vi "main(Test DQMH modules).bak.vi"() -> ()   [LabVIEW 2018, in "Application.lvlib"] (continued)
        n1621 = call "progress string(SubVI).vi"("String 3"=w3805, "String in"=w3806) -> ("String out"=w3807:string)  [unwired: 9 in]
        n1622 = call "FGV Driver Data.vi"("DUT index(1-60)"=w3804) -> ("DUT SC"=w3803:bool)  [unwired: 7 in, 3 out]
        n1623 = case shown="False" w3803 {
          tunnel: [w3832 _] -> w3812
          tunnel: w3809 -> [w3831 _]
          frame False {
            w3819 = T11 {"command"="", "command data"=variant} ("element")
            w3818 = "MEAS.mux6_1"
            n1624 = To Variant(anything=T4."mux6-1_channel0" ("mux6_1(3wires)_encode")) -> (Variant=w3817:variant)
            n1625 = To Variant(anything=T4."mux6_1_channel3_3" ("mux6_1(3wires)_encode")) -> (Variant=w3829:variant)
            n1626 = To Variant(anything=T4."mux6_1_channel3_2" ("mux6_1(3wires)_encode")) -> (Variant=w3827:variant)
            n1627 = Bundle By Name(cluster=w3819, "command"=w3818, "command data"=w3827) -> (w3826:T11)
            n1628 = Bundle By Name(cluster=w3819, "command"=w3818, "command data"=w3829) -> (w3825:T11)
            n1629 = Bundle By Name(cluster=w3819, "command"=w3818, "command data"=w3817) -> ()  [unwired: 1 out]
            n1630 = Bundle By Name(cluster=w3819, "command"="MEAS.DMM dual read") -> (w3823:T11)
            n1631 = Build Array(w3826, w3825, w3823) -> (w3821:T11[])
            n1632 = Reverse 1D Array(array=w3821) -> (reversed array=w3822:T11[])
            n1633 = for {
              tunnel: [w3838] -> w3832 mode=indexing
              tunnel: w3831 -> [w3837]
              tunnel: w3822 -> [w3836] mode=indexing
              n1634 = Unbundle By Name(w3836) -> ("command"=w3835:string, "command data"=w3834:variant)
              n1635 = call "App enquece.vi"("Priority Enquece"=TRUE, "command data"=w3834, "command"=w3835, "queue in"=w3837) -> ("error out"=w3838:errorcluster)  [unwired: 6 in, 1 out]
            }
          }
          frame True {
          }
        }
        n1636 = Merge Errors(w3810, w3812) -> (w3811:errorcluster)
      }
      frame "Test DRV 16" {
        w3845 = 16  # DUT index(0-59)
        n1637 = disable-structure shown="LOGGING==TRUE" {
          disable-tunnel: w3846 -> [w3881 _]
          frame condition #0 (active) {
            n1638 = Empty String/Path?(string/path=w3881) -> (empty?=w3884:bool)
            n1639 = Select(t="Quece timeout", s=w3884, f=w3881) -> (s? t:f=w3880:string)
            n1640 = call "string log (SubVI).vi"("Enum"=enum16{"Init", "Log", "Read"}."Log", "state Name"=w3880) -> ()  [unwired: 8 in, 2 out]
          }
          frame condition #1 {
          }
        }
        n1641 = call "progress string(SubVI).vi"("String 3"=w3846, "String in"=w3847) -> ("String out"=w3848:string)  [unwired: 9 in]
        n1642 = call "FGV Driver Data.vi"("DUT index(1-60)"=w3845) -> ("DUT SC"=w3844:bool)  [unwired: 7 in, 3 out]
        n1643 = case shown="False" w3844 {
          tunnel: [w3873 _] -> w3853
          tunnel: w3850 -> [w3872 _]
          frame False {
            w3860 = T11 {"command"="", "command data"=variant} ("element")
            w3859 = "MEAS.mux6_1"
            n1644 = To Variant(anything=T4."mux6-1_channel0" ("mux6_1(3wires)_encode")) -> (Variant=w3858:variant)
            n1645 = To Variant(anything=T4."mux6_1_channel4_3" ("mux6_1(3wires)_encode")) -> (Variant=w3870:variant)
            n1646 = To Variant(anything=T4."mux6_1_channel4_2" ("mux6_1(3wires)_encode")) -> (Variant=w3868:variant)
            n1647 = Bundle By Name(cluster=w3860, "command"=w3859, "command data"=w3868) -> (w3867:T11)
            n1648 = Bundle By Name(cluster=w3860, "command"=w3859, "command data"=w3870) -> (w3866:T11)
            n1649 = Bundle By Name(cluster=w3860, "command"=w3859, "command data"=w3858) -> ()  [unwired: 1 out]
            n1650 = Bundle By Name(cluster=w3860, "command"="MEAS.DMM dual read") -> (w3864:T11)
            n1651 = Build Array(w3867, w3866, w3864) -> (w3862:T11[])
            n1652 = Reverse 1D Array(array=w3862) -> (reversed array=w3863:T11[])
            n1653 = for {
              tunnel: [w3879] -> w3873 mode=indexing
              tunnel: w3872 -> [w3878]
              tunnel: w3863 -> [w3877] mode=indexing
              n1654 = Unbundle By Name(w3877) -> ("command"=w3876:string, "command data"=w3875:variant)
              n1655 = call "App enquece.vi"("Priority Enquece"=TRUE, "command data"=w3875, "command"=w3876, "queue in"=w3878) -> ("error out"=w3879:errorcluster)  [unwired: 6 in, 1 out]
            }
          }
          frame True {
          }
        }
        n1656 = Merge Errors(w3851, w3853) -> (w3852:errorcluster)
      }
      frame "Test DRV 17" {
        w3885 = 17  # DUT index(0-59)
        n1657 = disable-structure shown="LOGGING==TRUE" {
          disable-tunnel: w3887 -> [w3922 _]
          frame condition #0 (active) {
            n1658 = Empty String/Path?(string/path=w3922) -> (empty?=w3925:bool)
            n1659 = Select(t="Quece timeout", s=w3925, f=w3922) -> (s? t:f=w3921:string)
            n1660 = call "string log (SubVI).vi"("Enum"=enum16{"Init", "Log", "Read"}."Log", "state Name"=w3921) -> ()  [unwired: 8 in, 2 out]
          }
          frame condition #1 {
          }
        }
        n1661 = call "progress string(SubVI).vi"("String 3"=w3887, "String in"=w3888) -> ("String out"=w3889:string)  [unwired: 9 in]
        n1662 = call "FGV Driver Data.vi"("DUT index(1-60)"=w3885) -> ("DUT SC"=w3886:bool)  [unwired: 7 in, 3 out]
        n1663 = case shown="False" w3886 {
          tunnel: [w3914 _] -> w3894
          tunnel: w3891 -> [w3913 _]
          frame False {
            w3901 = T11 {"command"="", "command data"=variant} ("element")
            w3900 = "MEAS.mux6_1"
            n1664 = To Variant(anything=T4."mux6-1_channel0" ("mux6_1(3wires)_encode")) -> (Variant=w3899:variant)
            n1665 = To Variant(anything=T4."mux6_1_channel5_3" ("mux6_1(3wires)_encode")) -> (Variant=w3911:variant)
            n1666 = To Variant(anything=T4."mux6_1_channel5_2" ("mux6_1(3wires)_encode")) -> (Variant=w3909:variant)
            n1667 = Bundle By Name(cluster=w3901, "command"=w3900, "command data"=w3909) -> (w3908:T11)
            n1668 = Bundle By Name(cluster=w3901, "command"=w3900, "command data"=w3911) -> (w3907:T11)
            n1669 = Bundle By Name(cluster=w3901, "command"=w3900, "command data"=w3899) -> ()  [unwired: 1 out]
            n1670 = Bundle By Name(cluster=w3901, "command"="MEAS.DMM dual read") -> (w3905:T11)
            n1671 = Build Array(w3908, w3907, w3905) -> (w3903:T11[])
            n1672 = Reverse 1D Array(array=w3903) -> (reversed array=w3904:T11[])
            n1673 = for {
              tunnel: [w3920] -> w3914 mode=indexing
              tunnel: w3913 -> [w3919]
              tunnel: w3904 -> [w3918] mode=indexing
              n1674 = Unbundle By Name(w3918) -> ("command"=w3917:string, "command data"=w3916:variant)
              n1675 = call "App enquece.vi"("Priority Enquece"=TRUE, "command data"=w3916, "command"=w3917, "queue in"=w3919) -> ("error out"=w3920:errorcluster)  [unwired: 6 in, 1 out]
            }
          }
          frame True {
          }
        }
        n1676 = Merge Errors(w3892, w3894) -> (w3893:errorcluster)
      }
      frame "Test DRV 18" {
        w3929 = 18  # DUT index(0-59)
        n1677 = disable-structure shown="LOGGING==TRUE" {
          disable-tunnel: w3926 -> [w3963 _]
          frame condition #0 (active) {
            n1678 = Empty String/Path?(string/path=w3963) -> (empty?=w3966:bool)
            n1679 = Select(t="Quece timeout", s=w3966, f=w3963) -> (s? t:f=w3962:string)
            n1680 = call "string log (SubVI).vi"("Enum"=enum16{"Init", "Log", "Read"}."Log", "state Name"=w3962) -> ()  [unwired: 8 in, 2 out]
          }
          frame condition #1 {
          }
        }
        n1681 = call "progress string(SubVI).vi"("String 3"=w3926, "String in"=w3927) -> ("String out"=w3928:string)  [unwired: 9 in]
        n1682 = call "FGV Driver Data.vi"("DUT index(1-60)"=w3929) -> ("DUT SC"=w3930:bool)  [unwired: 7 in, 3 out]
        n1683 = case shown="False" w3930 {
          tunnel: [w3955 _] -> w3935
          tunnel: w3932 -> [w3954 _]
          frame False {
            w3942 = T11 {"command"="", "command data"=variant} ("element")
            w3941 = "MEAS.mux6_1"
            n1684 = To Variant(anything=T4."mux6-1_channel0" ("mux6_1(3wires)_encode")) -> (Variant=w3940:variant)
            n1685 = To Variant(anything=T4."mux6_1_channel6_3" ("mux6_1(3wires)_encode")) -> (Variant=w3952:variant)
            n1686 = To Variant(anything=T4."mux6_1_channel6_2" ("mux6_1(3wires)_encode")) -> (Variant=w3950:variant)
            n1687 = Bundle By Name(cluster=w3942, "command"=w3941, "command data"=w3950) -> (w3949:T11)
            n1688 = Bundle By Name(cluster=w3942, "command"=w3941, "command data"=w3952) -> (w3948:T11)
            n1689 = Bundle By Name(cluster=w3942, "command"=w3941, "command data"=w3940) -> ()  [unwired: 1 out]
            n1690 = Bundle By Name(cluster=w3942, "command"="MEAS.DMM dual read") -> (w3946:T11)
            n1691 = Build Array(w3949, w3948, w3946) -> (w3944:T11[])
            n1692 = Reverse 1D Array(array=w3944) -> (reversed array=w3945:T11[])
            n1693 = for {
              tunnel: [w3961] -> w3955 mode=indexing
              tunnel: w3954 -> [w3960]
              tunnel: w3945 -> [w3959] mode=indexing
              n1694 = Unbundle By Name(w3959) -> ("command"=w3958:string, "command data"=w3957:variant)
              n1695 = call "App enquece.vi"("Priority Enquece"=TRUE, "command data"=w3957, "command"=w3958, "queue in"=w3960) -> ("error out"=w3961:errorcluster)  [unwired: 6 in, 1 out]
            }
          }
          frame True {
          }
        }
        n1696 = Merge Errors(w3933, w3935) -> (w3934:errorcluster)
      }
      frame "Test DRV 19" {
        w3968 = 19  # DUT index(0-59)
        n1697 = disable-structure shown="LOGGING==TRUE" {
          disable-tunnel: w3969 -> [w4004 _]
          frame condition #0 (active) {
            n1698 = Empty String/Path?(string/path=w4004) -> (empty?=w4007:bool)
            n1699 = Select(t="Quece timeout", s=w4007, f=w4004) -> (s? t:f=w4003:string)
            n1700 = call "string log (SubVI).vi"("Enum"=enum16{"Init", "Log", "Read"}."Log", "state Name"=w4003) -> ()  [unwired: 8 in, 2 out]
          }
          frame condition #1 {
          }
        }
        n1701 = call "progress string(SubVI).vi"("String 3"=w3969, "String in"=w3970) -> ("String out"=w3971:string)  [unwired: 9 in]
        n1702 = call "FGV Driver Data.vi"("DUT index(1-60)"=w3968) -> ("DUT SC"=w3967:bool)  [unwired: 7 in, 3 out]
        n1703 = case shown="False" w3967 {
          tunnel: [w3996 _] -> w3976
          tunnel: w3973 -> [w3995 _]
          frame False {
            w3983 = T11 {"command"="", "command data"=variant} ("element")
            w3982 = "MEAS.mux6_1"
            n1704 = To Variant(anything=T4."mux6-1_channel0" ("mux6_1(3wires)_encode")) -> (Variant=w3981:variant)
            n1705 = To Variant(anything=T4."mux6_1_channel1_3" ("mux6_1(3wires)_encode")) -> (Variant=w3993:variant)
            n1706 = To Variant(anything=T4."mux6-1_channel1_2" ("mux6_1(3wires)_encode")) -> (Variant=w3991:variant)
            n1707 = Bundle By Name(cluster=w3983, "command"=w3982, "command data"=w3991) -> (w3990:T11)
            n1708 = Bundle By Name(cluster=w3983, "command"=w3982, "command data"=w3993) -> (w3989:T11)
            n1709 = Bundle By Name(cluster=w3983, "command"=w3982, "command data"=w3981) -> ()  [unwired: 1 out]
            n1710 = Bundle By Name(cluster=w3983, "command"="MEAS.DMM dual read") -> (w3987:T11)
            n1711 = Build Array(w3990, w3989, w3987) -> (w3985:T11[])
            n1712 = Reverse 1D Array(array=w3985) -> (reversed array=w3986:T11[])
            n1713 = for {
              tunnel: [w4002] -> w3996 mode=indexing
              tunnel: w3995 -> [w4001]
              tunnel: w3986 -> [w4000] mode=indexing
              n1714 = Unbundle By Name(w4000) -> ("command"=w3999:string, "command data"=w3998:variant)
              n1715 = call "App enquece.vi"("Priority Enquece"=TRUE, "command data"=w3998, "command"=w3999, "queue in"=w4001) -> ("error out"=w4002:errorcluster)  [unwired: 6 in, 1 out]
            }
          }
          frame True {
          }
        }
        n1716 = Merge Errors(w3974, w3976) -> (w3975:errorcluster)
      }
      frame "Test DRV 20" {
        w4009 = 20  # DUT index(0-59)
        n1717 = disable-structure shown="LOGGING==TRUE" {
          disable-tunnel: w4010 -> [w4045 _]
          frame condition #0 (active) {
            n1718 = Empty String/Path?(string/path=w4045) -> (empty?=w4048:bool)
            n1719 = Select(t="Quece timeout", s=w4048, f=w4045) -> (s? t:f=w4044:string)
            n1720 = call "string log (SubVI).vi"("Enum"=enum16{"Init", "Log", "Read"}."Log", "state Name"=w4044) -> ()  [unwired: 8 in, 2 out]
          }
          frame condition #1 {
          }
        }
        n1721 = call "progress string(SubVI).vi"("String 3"=w4010, "String in"=w4011) -> ("String out"=w4012:string)  [unwired: 9 in]
        n1722 = call "FGV Driver Data.vi"("DUT index(1-60)"=w4009) -> ("DUT SC"=w4008:bool)  [unwired: 7 in, 3 out]
        n1723 = case shown="False" w4008 {
          tunnel: [w4037 _] -> w4017
          tunnel: w4014 -> [w4036 _]
          frame False {
            w4024 = T11 {"command"="", "command data"=variant} ("element")
            w4023 = "MEAS.mux6_1"
            n1724 = To Variant(anything=T4."mux6-1_channel0" ("mux6_1(3wires)_encode")) -> (Variant=w4022:variant)
            n1725 = To Variant(anything=T4."mux6_1_channel2_3" ("mux6_1(3wires)_encode")) -> (Variant=w4034:variant)
            n1726 = To Variant(anything=T4."mux6_1_channel2_2" ("mux6_1(3wires)_encode")) -> (Variant=w4032:variant)
            n1727 = Bundle By Name(cluster=w4024, "command"=w4023, "command data"=w4032) -> (w4031:T11)
            n1728 = Bundle By Name(cluster=w4024, "command"=w4023, "command data"=w4034) -> (w4030:T11)
            n1729 = Bundle By Name(cluster=w4024, "command"=w4023, "command data"=w4022) -> ()  [unwired: 1 out]
            n1730 = Bundle By Name(cluster=w4024, "command"="MEAS.DMM dual read") -> (w4028:T11)
            n1731 = Build Array(w4031, w4030, w4028) -> (w4026:T11[])
            n1732 = Reverse 1D Array(array=w4026) -> (reversed array=w4027:T11[])
            n1733 = for {
              tunnel: [w4043] -> w4037 mode=indexing
              tunnel: w4036 -> [w4042]
              tunnel: w4027 -> [w4041] mode=indexing
              n1734 = Unbundle By Name(w4041) -> ("command"=w4040:string, "command data"=w4039:variant)
              n1735 = call "App enquece.vi"("Priority Enquece"=TRUE, "command data"=w4039, "command"=w4040, "queue in"=w4042) -> ("error out"=w4043:errorcluster)  [unwired: 6 in, 1 out]
            }
          }
          frame True {
          }
        }
        n1736 = Merge Errors(w4015, w4017) -> (w4016:errorcluster)
      }
      frame "Test DRV 21" {
        w4050 = 21  # DUT index(0-59)
        n1737 = disable-structure shown="LOGGING==TRUE" {
          disable-tunnel: w4051 -> [w4086 _]
          frame condition #0 (active) {
            n1738 = Empty String/Path?(string/path=w4086) -> (empty?=w4089:bool)
            n1739 = Select(t="Quece timeout", s=w4089, f=w4086) -> (s? t:f=w4085:string)
            n1740 = call "string log (SubVI).vi"("Enum"=enum16{"Init", "Log", "Read"}."Log", "state Name"=w4085) -> ()  [unwired: 8 in, 2 out]
          }
          frame condition #1 {
          }
        }
        n1741 = call "progress string(SubVI).vi"("String 3"=w4051, "String in"=w4052) -> ("String out"=w4053:string)  [unwired: 9 in]
        n1742 = call "FGV Driver Data.vi"("DUT index(1-60)"=w4050) -> ("DUT SC"=w4049:bool)  [unwired: 7 in, 3 out]
        n1743 = case shown="False" w4049 {
          tunnel: [w4078 _] -> w4058
          tunnel: w4055 -> [w4077 _]
          frame False {
            w4065 = T11 {"command"="", "command data"=variant} ("element")
            w4064 = "MEAS.mux6_1"
            n1744 = To Variant(anything=T4."mux6-1_channel0" ("mux6_1(3wires)_encode")) -> (Variant=w4063:variant)
            n1745 = To Variant(anything=T4."mux6_1_channel3_3" ("mux6_1(3wires)_encode")) -> (Variant=w4075:variant)
            n1746 = To Variant(anything=T4."mux6_1_channel3_2" ("mux6_1(3wires)_encode")) -> (Variant=w4073:variant)
            n1747 = Bundle By Name(cluster=w4065, "command"=w4064, "command data"=w4073) -> (w4072:T11)
            n1748 = Bundle By Name(cluster=w4065, "command"=w4064, "command data"=w4075) -> (w4071:T11)
            n1749 = Bundle By Name(cluster=w4065, "command"=w4064, "command data"=w4063) -> ()  [unwired: 1 out]
            n1750 = Bundle By Name(cluster=w4065, "command"="MEAS.DMM dual read") -> (w4069:T11)
            n1751 = Build Array(w4072, w4071, w4069) -> (w4067:T11[])
            n1752 = Reverse 1D Array(array=w4067) -> (reversed array=w4068:T11[])
            n1753 = for {
              tunnel: [w4084] -> w4078 mode=indexing
              tunnel: w4077 -> [w4083]
              tunnel: w4068 -> [w4082] mode=indexing
              n1754 = Unbundle By Name(w4082) -> ("command"=w4081:string, "command data"=w4080:variant)
              n1755 = call "App enquece.vi"("Priority Enquece"=TRUE, "command data"=w4080, "command"=w4081, "queue in"=w4083) -> ("error out"=w4084:errorcluster)  [unwired: 6 in, 1 out]
            }
          }
          frame True {
          }
        }
        n1756 = Merge Errors(w4056, w4058) -> (w4057:errorcluster)
      }
      frame "Test DRV 22" {
        w4091 = 22  # DUT index(0-59)
        n1757 = disable-structure shown="LOGGING==TRUE" {
          disable-tunnel: w4092 -> [w4127 _]
          frame condition #0 (active) {
            n1758 = Empty String/Path?(string/path=w4127) -> (empty?=w4130:bool)
            n1759 = Select(t="Quece timeout", s=w4130, f=w4127) -> (s? t:f=w4126:string)
            n1760 = call "string log (SubVI).vi"("Enum"=enum16{"Init", "Log", "Read"}."Log", "state Name"=w4126) -> ()  [unwired: 8 in, 2 out]
          }
          frame condition #1 {
          }
        }
        n1761 = call "progress string(SubVI).vi"("String 3"=w4092, "String in"=w4093) -> ("String out"=w4094:string)  [unwired: 9 in]
        n1762 = call "FGV Driver Data.vi"("DUT index(1-60)"=w4091) -> ("DUT SC"=w4090:bool)  [unwired: 7 in, 3 out]
        n1763 = case shown="False" w4090 {
          tunnel: [w4119 _] -> w4099
          tunnel: w4096 -> [w4118 _]
          frame False {
            w4106 = T11 {"command"="", "command data"=variant} ("element")
            w4105 = "MEAS.mux6_1"
            n1764 = To Variant(anything=T4."mux6-1_channel0" ("mux6_1(3wires)_encode")) -> (Variant=w4104:variant)
            n1765 = To Variant(anything=T4."mux6_1_channel4_3" ("mux6_1(3wires)_encode")) -> (Variant=w4116:variant)
            n1766 = To Variant(anything=T4."mux6_1_channel4_2" ("mux6_1(3wires)_encode")) -> (Variant=w4114:variant)
            n1767 = Bundle By Name(cluster=w4106, "command"=w4105, "command data"=w4114) -> (w4113:T11)
            n1768 = Bundle By Name(cluster=w4106, "command"=w4105, "command data"=w4116) -> (w4112:T11)
            n1769 = Bundle By Name(cluster=w4106, "command"=w4105, "command data"=w4104) -> ()  [unwired: 1 out]
            n1770 = Bundle By Name(cluster=w4106, "command"="MEAS.DMM dual read") -> (w4110:T11)
            n1771 = Build Array(w4113, w4112, w4110) -> (w4108:T11[])
            n1772 = Reverse 1D Array(array=w4108) -> (reversed array=w4109:T11[])
            n1773 = for {
              tunnel: [w4125] -> w4119 mode=indexing
              tunnel: w4118 -> [w4124]
              tunnel: w4109 -> [w4123] mode=indexing
              n1774 = Unbundle By Name(w4123) -> ("command"=w4122:string, "command data"=w4121:variant)
              n1775 = call "App enquece.vi"("Priority Enquece"=TRUE, "command data"=w4121, "command"=w4122, "queue in"=w4124) -> ("error out"=w4125:errorcluster)  [unwired: 6 in, 1 out]
            }
          }
          frame True {
          }
        }
        n1776 = Merge Errors(w4097, w4099) -> (w4098:errorcluster)
      }
      frame "Test DRV 23" {
        w4132 = 23  # DUT index(0-59)
        n1777 = disable-structure shown="LOGGING==TRUE" {
          disable-tunnel: w4133 -> [w4168 _]
          frame condition #0 (active) {
            n1778 = Empty String/Path?(string/path=w4168) -> (empty?=w4171:bool)
            n1779 = Select(t="Quece timeout", s=w4171, f=w4168) -> (s? t:f=w4167:string)
            n1780 = call "string log (SubVI).vi"("Enum"=enum16{"Init", "Log", "Read"}."Log", "state Name"=w4167) -> ()  [unwired: 8 in, 2 out]
          }
          frame condition #1 {
          }
        }
        n1781 = call "progress string(SubVI).vi"("String 3"=w4133, "String in"=w4134) -> ("String out"=w4135:string)  [unwired: 9 in]
        n1782 = call "FGV Driver Data.vi"("DUT index(1-60)"=w4132) -> ("DUT SC"=w4131:bool)  [unwired: 7 in, 3 out]
        n1783 = case shown="False" w4131 {
          tunnel: [w4160 _] -> w4140
          tunnel: w4137 -> [w4159 _]
          frame False {
            w4147 = T11 {"command"="", "command data"=variant} ("element")
            w4146 = "MEAS.mux6_1"
            n1784 = To Variant(anything=T4."mux6-1_channel0" ("mux6_1(3wires)_encode")) -> (Variant=w4145:variant)
            n1785 = To Variant(anything=T4."mux6_1_channel5_3" ("mux6_1(3wires)_encode")) -> (Variant=w4157:variant)
            n1786 = To Variant(anything=T4."mux6_1_channel5_2" ("mux6_1(3wires)_encode")) -> (Variant=w4155:variant)
            n1787 = Bundle By Name(cluster=w4147, "command"=w4146, "command data"=w4155) -> (w4154:T11)
            n1788 = Bundle By Name(cluster=w4147, "command"=w4146, "command data"=w4157) -> (w4153:T11)
            n1789 = Bundle By Name(cluster=w4147, "command"=w4146, "command data"=w4145) -> ()  [unwired: 1 out]
            n1790 = Bundle By Name(cluster=w4147, "command"="MEAS.DMM dual read") -> (w4151:T11)
            n1791 = Build Array(w4154, w4153, w4151) -> (w4149:T11[])
            n1792 = Reverse 1D Array(array=w4149) -> (reversed array=w4150:T11[])
            n1793 = for {
              tunnel: [w4166] -> w4160 mode=indexing
              tunnel: w4159 -> [w4165]
              tunnel: w4150 -> [w4164] mode=indexing
              n1794 = Unbundle By Name(w4164) -> ("command"=w4163:string, "command data"=w4162:variant)
              n1795 = call "App enquece.vi"("Priority Enquece"=TRUE, "command data"=w4162, "command"=w4163, "queue in"=w4165) -> ("error out"=w4166:errorcluster)  [unwired: 6 in, 1 out]
            }
          }
          frame True {
          }
        }
        n1796 = Merge Errors(w4138, w4140) -> (w4139:errorcluster)
      }
      frame "Test DRV 24" {
        w4173 = 24  # DUT index(0-59)
        n1797 = disable-structure shown="LOGGING==TRUE" {
          disable-tunnel: w4174 -> [w4209 _]
          frame condition #0 (active) {
            n1798 = Empty String/Path?(string/path=w4209) -> (empty?=w4212:bool)
            n1799 = Select(t="Quece timeout", s=w4212, f=w4209) -> (s? t:f=w4208:string)
            n1800 = call "string log (SubVI).vi"("Enum"=enum16{"Init", "Log", "Read"}."Log", "state Name"=w4208) -> ()  [unwired: 8 in, 2 out]
          }
          frame condition #1 {
          }
        }
        n1801 = call "progress string(SubVI).vi"("String 3"=w4174, "String in"=w4175) -> ("String out"=w4176:string)  [unwired: 9 in]
        n1802 = call "FGV Driver Data.vi"("DUT index(1-60)"=w4173) -> ("DUT SC"=w4172:bool)  [unwired: 7 in, 3 out]
        n1803 = case shown="False" w4172 {
          tunnel: [w4201 _] -> w4181
          tunnel: w4178 -> [w4200 _]
          frame False {
            w4188 = T11 {"command"="", "command data"=variant} ("element")
            w4187 = "MEAS.mux6_1"
            n1804 = To Variant(anything=T4."mux6-1_channel0" ("mux6_1(3wires)_encode")) -> (Variant=w4186:variant)
            n1805 = To Variant(anything=T4."mux6_1_channel6_3" ("mux6_1(3wires)_encode")) -> (Variant=w4198:variant)
            n1806 = To Variant(anything=T4."mux6_1_channel6_2" ("mux6_1(3wires)_encode")) -> (Variant=w4196:variant)
            n1807 = Bundle By Name(cluster=w4188, "command"=w4187, "command data"=w4196) -> (w4195:T11)
            n1808 = Bundle By Name(cluster=w4188, "command"=w4187, "command data"=w4198) -> (w4194:T11)
            n1809 = Bundle By Name(cluster=w4188, "command"=w4187, "command data"=w4186) -> ()  [unwired: 1 out]
            n1810 = Bundle By Name(cluster=w4188, "command"="MEAS.DMM dual read") -> (w4192:T11)
            n1811 = Build Array(w4195, w4194, w4192) -> (w4190:T11[])
            n1812 = Reverse 1D Array(array=w4190) -> (reversed array=w4191:T11[])
            n1813 = for {
              tunnel: [w4207] -> w4201 mode=indexing
              tunnel: w4200 -> [w4206]
              tunnel: w4191 -> [w4205] mode=indexing
              n1814 = Unbundle By Name(w4205) -> ("command"=w4204:string, "command data"=w4203:variant)
              n1815 = call "App enquece.vi"("Priority Enquece"=TRUE, "command data"=w4203, "command"=w4204, "queue in"=w4206) -> ("error out"=w4207:errorcluster)  [unwired: 6 in, 1 out]
            }
          }
          frame True {
          }
        }
        n1816 = Merge Errors(w4179, w4181) -> (w4180:errorcluster)
      }
      frame "Test DRV 25" {
        w4214 = 25  # DUT index(0-59)
        n1817 = disable-structure shown="LOGGING==TRUE" {
          disable-tunnel: w4215 -> [w4250 _]
          frame condition #0 (active) {
            n1818 = Empty String/Path?(string/path=w4250) -> (empty?=w4253:bool)
            n1819 = Select(t="Quece timeout", s=w4253, f=w4250) -> (s? t:f=w4249:string)
            n1820 = call "string log (SubVI).vi"("Enum"=enum16{"Init", "Log", "Read"}."Log", "state Name"=w4249) -> ()  [unwired: 8 in, 2 out]
          }
          frame condition #1 {
          }
        }
        n1821 = call "progress string(SubVI).vi"("String 3"=w4215, "String in"=w4216) -> ("String out"=w4217:string)  [unwired: 9 in]
        n1822 = call "FGV Driver Data.vi"("DUT index(1-60)"=w4214) -> ("DUT SC"=w4213:bool)  [unwired: 7 in, 3 out]
        n1823 = case shown="False" w4213 {
          tunnel: [w4242 _] -> w4222
          tunnel: w4219 -> [w4241 _]
          frame False {
            w4229 = T11 {"command"="", "command data"=variant} ("element")
            w4228 = "MEAS.mux6_1"
            n1824 = To Variant(anything=T4."mux6-1_channel0" ("mux6_1(3wires)_encode")) -> (Variant=w4227:variant)
            n1825 = To Variant(anything=T4."mux6_1_channel1_3" ("mux6_1(3wires)_encode")) -> (Variant=w4239:variant)
            n1826 = To Variant(anything=T4."mux6-1_channel1_2" ("mux6_1(3wires)_encode")) -> (Variant=w4237:variant)
            n1827 = Bundle By Name(cluster=w4229, "command"=w4228, "command data"=w4237) -> (w4236:T11)
            n1828 = Bundle By Name(cluster=w4229, "command"=w4228, "command data"=w4239) -> (w4235:T11)
            n1829 = Bundle By Name(cluster=w4229, "command"=w4228, "command data"=w4227) -> ()  [unwired: 1 out]
            n1830 = Bundle By Name(cluster=w4229, "command"="MEAS.DMM dual read") -> (w4233:T11)
            n1831 = Build Array(w4236, w4235, w4233) -> (w4231:T11[])
            n1832 = Reverse 1D Array(array=w4231) -> (reversed array=w4232:T11[])
            n1833 = for {
              tunnel: [w4248] -> w4242 mode=indexing
              tunnel: w4241 -> [w4247]
              tunnel: w4232 -> [w4246] mode=indexing
              n1834 = Unbundle By Name(w4246) -> ("command"=w4245:string, "command data"=w4244:variant)
              n1835 = call "App enquece.vi"("Priority Enquece"=TRUE, "command data"=w4244, "command"=w4245, "queue in"=w4247) -> ("error out"=w4248:errorcluster)  [unwired: 6 in, 1 out]
            }
          }
          frame True {
          }
        }
        n1836 = Merge Errors(w4220, w4222) -> (w4221:errorcluster)
      }
      frame "Test DRV 26" {
        w4255 = 26  # DUT index(0-59)
        n1837 = disable-structure shown="LOGGING==TRUE" {
          disable-tunnel: w4256 -> [w4291 _]
          frame condition #0 (active) {
            n1838 = Empty String/Path?(string/path=w4291) -> (empty?=w4294:bool)
            n1839 = Select(t="Quece timeout", s=w4294, f=w4291) -> (s? t:f=w4290:string)
            n1840 = call "string log (SubVI).vi"("Enum"=enum16{"Init", "Log", "Read"}."Log", "state Name"=w4290) -> ()  [unwired: 8 in, 2 out]
          }
          frame condition #1 {
          }
        }
        n1841 = call "progress string(SubVI).vi"("String 3"=w4256, "String in"=w4257) -> ("String out"=w4258:string)  [unwired: 9 in]
        n1842 = call "FGV Driver Data.vi"("DUT index(1-60)"=w4255) -> ("DUT SC"=w4254:bool)  [unwired: 7 in, 3 out]
        n1843 = case shown="False" w4254 {
          tunnel: [w4283 _] -> w4263
          tunnel: w4260 -> [w4282 _]
          frame False {
            w4270 = T11 {"command"="", "command data"=variant} ("element")
            w4269 = "MEAS.mux6_1"
            n1844 = To Variant(anything=T4."mux6-1_channel0" ("mux6_1(3wires)_encode")) -> (Variant=w4268:variant)
            n1845 = To Variant(anything=T4."mux6_1_channel2_3" ("mux6_1(3wires)_encode")) -> (Variant=w4280:variant)
            n1846 = To Variant(anything=T4."mux6_1_channel2_2" ("mux6_1(3wires)_encode")) -> (Variant=w4278:variant)
            n1847 = Bundle By Name(cluster=w4270, "command"=w4269, "command data"=w4278) -> (w4277:T11)
            n1848 = Bundle By Name(cluster=w4270, "command"=w4269, "command data"=w4280) -> (w4276:T11)
            n1849 = Bundle By Name(cluster=w4270, "command"=w4269, "command data"=w4268) -> ()  [unwired: 1 out]
            n1850 = Bundle By Name(cluster=w4270, "command"="MEAS.DMM dual read") -> (w4274:T11)
            n1851 = Build Array(w4277, w4276, w4274) -> (w4272:T11[])
            n1852 = Reverse 1D Array(array=w4272) -> (reversed array=w4273:T11[])
            n1853 = for {
              tunnel: [w4289] -> w4283 mode=indexing
              tunnel: w4282 -> [w4288]
              tunnel: w4273 -> [w4287] mode=indexing
              n1854 = Unbundle By Name(w4287) -> ("command"=w4286:string, "command data"=w4285:variant)
              n1855 = call "App enquece.vi"("Priority Enquece"=TRUE, "command data"=w4285, "command"=w4286, "queue in"=w4288) -> ("error out"=w4289:errorcluster)  [unwired: 6 in, 1 out]
            }
          }
          frame True {
          }
        }
        n1856 = Merge Errors(w4261, w4263) -> (w4262:errorcluster)
      }
      frame "Test DRV 27" {
        w4296 = 27  # DUT index(0-59)
        n1857 = disable-structure shown="LOGGING==TRUE" {
          disable-tunnel: w4297 -> [w4332 _]
          frame condition #0 (active) {
            n1858 = Empty String/Path?(string/path=w4332) -> (empty?=w4335:bool)
            n1859 = Select(t="Quece timeout", s=w4335, f=w4332) -> (s? t:f=w4331:string)
            n1860 = call "string log (SubVI).vi"("Enum"=enum16{"Init", "Log", "Read"}."Log", "state Name"=w4331) -> ()  [unwired: 8 in, 2 out]
          }
          frame condition #1 {
          }
        }
        n1861 = call "progress string(SubVI).vi"("String 3"=w4297, "String in"=w4298) -> ("String out"=w4299:string)  [unwired: 9 in]
        n1862 = call "FGV Driver Data.vi"("DUT index(1-60)"=w4296) -> ("DUT SC"=w4295:bool)  [unwired: 7 in, 3 out]
        n1863 = case shown="False" w4295 {
          tunnel: [w4324 _] -> w4304
          tunnel: w4301 -> [w4323 _]
          frame False {
            w4311 = T11 {"command"="", "command data"=variant} ("element")
            w4310 = "MEAS.mux6_1"
            n1864 = To Variant(anything=T4."mux6-1_channel0" ("mux6_1(3wires)_encode")) -> (Variant=w4309:variant)
            n1865 = To Variant(anything=T4."mux6_1_channel3_3" ("mux6_1(3wires)_encode")) -> (Variant=w4321:variant)
            n1866 = To Variant(anything=T4."mux6_1_channel3_2" ("mux6_1(3wires)_encode")) -> (Variant=w4319:variant)
            n1867 = Bundle By Name(cluster=w4311, "command"=w4310, "command data"=w4319) -> (w4318:T11)
            n1868 = Bundle By Name(cluster=w4311, "command"=w4310, "command data"=w4321) -> (w4317:T11)
            n1869 = Bundle By Name(cluster=w4311, "command"=w4310, "command data"=w4309) -> ()  [unwired: 1 out]
            n1870 = Bundle By Name(cluster=w4311, "command"="MEAS.DMM dual read") -> (w4315:T11)
            n1871 = Build Array(w4318, w4317, w4315) -> (w4313:T11[])
            n1872 = Reverse 1D Array(array=w4313) -> (reversed array=w4314:T11[])
            n1873 = for {
              tunnel: [w4330] -> w4324 mode=indexing
              tunnel: w4323 -> [w4329]
              tunnel: w4314 -> [w4328] mode=indexing
              n1874 = Unbundle By Name(w4328) -> ("command"=w4327:string, "command data"=w4326:variant)
              n1875 = call "App enquece.vi"("Priority Enquece"=TRUE, "command data"=w4326, "command"=w4327, "queue in"=w4329) -> ("error out"=w4330:errorcluster)  [unwired: 6 in, 1 out]
            }
          }
          frame True {
          }
        }
        n1876 = Merge Errors(w4302, w4304) -> (w4303:errorcluster)
      }
      frame "Test DRV 28" {
        w4337 = 28  # DUT index(0-59)
        n1877 = disable-structure shown="LOGGING==TRUE" {
          disable-tunnel: w4338 -> [w4373 _]
          frame condition #0 (active) {
            n1878 = Empty String/Path?(string/path=w4373) -> (empty?=w4376:bool)
            n1879 = Select(t="Quece timeout", s=w4376, f=w4373) -> (s? t:f=w4372:string)
            n1880 = call "string log (SubVI).vi"("Enum"=enum16{"Init", "Log", "Read"}."Log", "state Name"=w4372) -> ()  [unwired: 8 in, 2 out]
          }
          frame condition #1 {
          }
        }
        n1881 = call "progress string(SubVI).vi"("String 3"=w4338, "String in"=w4339) -> ("String out"=w4340:string)  [unwired: 9 in]
        n1882 = call "FGV Driver Data.vi"("DUT index(1-60)"=w4337) -> ("DUT SC"=w4336:bool)  [unwired: 7 in, 3 out]
        n1883 = case shown="False" w4336 {
          tunnel: [w4365 _] -> w4345
          tunnel: w4342 -> [w4364 _]
          frame False {
            w4350 = T11 {"command"="", "command data"=variant} ("element")
            w4352 = "MEAS.mux6_1"
            n1884 = To Variant(anything=T4."mux6-1_channel0" ("mux6_1(3wires)_encode")) -> (Variant=w4351:variant)
            n1885 = To Variant(anything=T4."mux6_1_channel4_3" ("mux6_1(3wires)_encode")) -> (Variant=w4362:variant)
            n1886 = To Variant(anything=T4."mux6_1_channel4_2" ("mux6_1(3wires)_encode")) -> (Variant=w4360:variant)
            n1887 = Bundle By Name(cluster=w4350, "command"=w4352, "command data"=w4360) -> (w4359:T11)
            n1888 = Bundle By Name(cluster=w4350, "command"=w4352, "command data"=w4362) -> (w4358:T11)
            n1889 = Bundle By Name(cluster=w4350, "command"=w4352, "command data"=w4351) -> ()  [unwired: 1 out]
            n1890 = Bundle By Name(cluster=w4350, "command"="MEAS.DMM dual read") -> (w4356:T11)
            n1891 = Build Array(w4359, w4358, w4356) -> (w4354:T11[])
            n1892 = Reverse 1D Array(array=w4354) -> (reversed array=w4355:T11[])
            n1893 = for {
              tunnel: [w4371] -> w4365 mode=indexing
              tunnel: w4364 -> [w4370]
              tunnel: w4355 -> [w4369] mode=indexing
              n1894 = Unbundle By Name(w4369) -> ("command"=w4368:string, "command data"=w4367:variant)
              n1895 = call "App enquece.vi"("Priority Enquece"=TRUE, "command data"=w4367, "command"=w4368, "queue in"=w4370) -> ("error out"=w4371:errorcluster)  [unwired: 6 in, 1 out]
            }
          }
          frame True {
          }
        }
        n1896 = Merge Errors(w4343, w4345) -> (w4344:errorcluster)
      }
      frame "Test DRV 29" {
        w4378 = 29  # DUT index(0-59)
        n1897 = disable-structure shown="LOGGING==TRUE" {
          disable-tunnel: w4379 -> [w4414 _]
          frame condition #0 (active) {
            n1898 = Empty String/Path?(string/path=w4414) -> (empty?=w4417:bool)
            n1899 = Select(t="Quece timeout", s=w4417, f=w4414) -> (s? t:f=w4413:string)
            n1900 = call "string log (SubVI).vi"("Enum"=enum16{"Init", "Log", "Read"}."Log", "state Name"=w4413) -> ()  [unwired: 8 in, 2 out]
          }
          frame condition #1 {
          }
        }
        n1901 = call "progress string(SubVI).vi"("String 3"=w4379, "String in"=w4380) -> ("String out"=w4381:string)  [unwired: 9 in]
        n1902 = call "FGV Driver Data.vi"("DUT index(1-60)"=w4378) -> ("DUT SC"=w4377:bool)  [unwired: 7 in, 3 out]
        n1903 = case shown="False" w4377 {
          tunnel: [w4406 _] -> w4386
          tunnel: w4383 -> [w4405 _]
          frame False {
            w4393 = T11 {"command"="", "command data"=variant} ("element")
            w4392 = "MEAS.mux6_1"
            n1904 = To Variant(anything=T4."mux6-1_channel0" ("mux6_1(3wires)_encode")) -> (Variant=w4391:variant)
            n1905 = To Variant(anything=T4."mux6_1_channel5_3" ("mux6_1(3wires)_encode")) -> (Variant=w4403:variant)
            n1906 = To Variant(anything=T4."mux6_1_channel5_2" ("mux6_1(3wires)_encode")) -> (Variant=w4401:variant)
            n1907 = Bundle By Name(cluster=w4393, "command"=w4392, "command data"=w4401) -> (w4400:T11)
            n1908 = Bundle By Name(cluster=w4393, "command"=w4392, "command data"=w4403) -> (w4399:T11)
            n1909 = Bundle By Name(cluster=w4393, "command"=w4392, "command data"=w4391) -> ()  [unwired: 1 out]
            n1910 = Bundle By Name(cluster=w4393, "command"="MEAS.DMM dual read") -> (w4397:T11)
            n1911 = Build Array(w4400, w4399, w4397) -> (w4395:T11[])
            n1912 = Reverse 1D Array(array=w4395) -> (reversed array=w4396:T11[])
            n1913 = for {
              tunnel: [w4412] -> w4406 mode=indexing
              tunnel: w4405 -> [w4411]
              tunnel: w4396 -> [w4410] mode=indexing
              n1914 = Unbundle By Name(w4410) -> ("command"=w4409:string, "command data"=w4408:variant)
              n1915 = call "App enquece.vi"("Priority Enquece"=TRUE, "command data"=w4408, "command"=w4409, "queue in"=w4411) -> ("error out"=w4412:errorcluster)  [unwired: 6 in, 1 out]
            }
          }
          frame True {
          }
        }
        n1916 = Merge Errors(w4384, w4386) -> (w4385:errorcluster)
      }
      frame "Test DRV 30" {
        w4418 = 30  # DUT index(0-59)
        n1917 = disable-structure shown="LOGGING==TRUE" {
          disable-tunnel: w4420 -> [w4455 _]
          frame condition #0 (active) {
            n1918 = Empty String/Path?(string/path=w4455) -> (empty?=w4458:bool)
            n1919 = Select(t="Quece timeout", s=w4458, f=w4455) -> (s? t:f=w4454:string)
            n1920 = call "string log (SubVI).vi"("Enum"=enum16{"Init", "Log", "Read"}."Log", "state Name"=w4454) -> ()  [unwired: 8 in, 2 out]
          }
          frame condition #1 {
          }
        }
        n1921 = call "progress string(SubVI).vi"("String 3"=w4420, "String in"=w4421) -> ("String out"=w4422:string)  [unwired: 9 in]
        n1922 = call "FGV Driver Data.vi"("DUT index(1-60)"=w4418) -> ("DUT SC"=w4419:bool)  [unwired: 7 in, 3 out]
        n1923 = case shown="False" w4419 {
          tunnel: [w4447 _] -> w4427
          tunnel: w4424 -> [w4446 _]
          frame False {
            w4434 = T11 {"command"="", "command data"=variant} ("element")
            w4433 = "MEAS.mux6_1"
            n1924 = To Variant(anything=T4."mux6-1_channel0" ("mux6_1(3wires)_encode")) -> (Variant=w4432:variant)
            n1925 = To Variant(anything=T4."mux6_1_channel6_3" ("mux6_1(3wires)_encode")) -> (Variant=w4444:variant)
            n1926 = To Variant(anything=T4."mux6_1_channel6_2" ("mux6_1(3wires)_encode")) -> (Variant=w4442:variant)
            n1927 = Bundle By Name(cluster=w4434, "command"=w4433, "command data"=w4442) -> (w4441:T11)
            n1928 = Bundle By Name(cluster=w4434, "command"=w4433, "command data"=w4444) -> (w4440:T11)
            n1929 = Bundle By Name(cluster=w4434, "command"=w4433, "command data"=w4432) -> ()  [unwired: 1 out]
            n1930 = Bundle By Name(cluster=w4434, "command"="MEAS.DMM dual read") -> (w4438:T11)
            n1931 = Build Array(w4441, w4440, w4438) -> (w4436:T11[])
            n1932 = Reverse 1D Array(array=w4436) -> (reversed array=w4437:T11[])
            n1933 = for {
              tunnel: [w4453] -> w4447 mode=indexing
              tunnel: w4446 -> [w4452]
              tunnel: w4437 -> [w4451] mode=indexing
              n1934 = Unbundle By Name(w4451) -> ("command"=w4450:string, "command data"=w4449:variant)
              n1935 = call "App enquece.vi"("Priority Enquece"=TRUE, "command data"=w4449, "command"=w4450, "queue in"=w4452) -> ("error out"=w4453:errorcluster)  [unwired: 6 in, 1 out]
            }
          }
          frame True {
          }
        }
        n1936 = Merge Errors(w4425, w4427) -> (w4426:errorcluster)
      }
      frame "Test DRV 31" {
        w4460 = 31  # DUT index(0-59)
        n1937 = disable-structure shown="LOGGING==TRUE" {
          disable-tunnel: w4461 -> [w4496 _]
          frame condition #0 (active) {
            n1938 = Empty String/Path?(string/path=w4496) -> (empty?=w4499:bool)
            n1939 = Select(t="Quece timeout", s=w4499, f=w4496) -> (s? t:f=w4495:string)
            n1940 = call "string log (SubVI).vi"("Enum"=enum16{"Init", "Log", "Read"}."Log", "state Name"=w4495) -> ()  [unwired: 8 in, 2 out]
          }
          frame condition #1 {
          }
        }
        n1941 = call "progress string(SubVI).vi"("String 3"=w4461, "String in"=w4462) -> ("String out"=w4463:string)  [unwired: 9 in]
        n1942 = call "FGV Driver Data.vi"("DUT index(1-60)"=w4460) -> ("DUT SC"=w4459:bool)  [unwired: 7 in, 3 out]
        n1943 = case shown="False" w4459 {
          tunnel: [w4488 _] -> w4468
          tunnel: w4465 -> [w4487 _]
          frame False {
            w4475 = T11 {"command"="", "command data"=variant} ("element")
            w4474 = "MEAS.mux6_1"
            n1944 = To Variant(anything=T4."mux6-1_channel0" ("mux6_1(3wires)_encode")) -> (Variant=w4473:variant)
            n1945 = To Variant(anything=T4."mux6_1_channel1_3" ("mux6_1(3wires)_encode")) -> (Variant=w4485:variant)
            n1946 = To Variant(anything=T4."mux6-1_channel1_2" ("mux6_1(3wires)_encode")) -> (Variant=w4483:variant)
            n1947 = Bundle By Name(cluster=w4475, "command"=w4474, "command data"=w4483) -> (w4482:T11)
            n1948 = Bundle By Name(cluster=w4475, "command"=w4474, "command data"=w4485) -> (w4481:T11)
            n1949 = Bundle By Name(cluster=w4475, "command"=w4474, "command data"=w4473) -> ()  [unwired: 1 out]
            n1950 = Bundle By Name(cluster=w4475, "command"="MEAS.DMM dual read") -> (w4479:T11)
            n1951 = Build Array(w4482, w4481, w4479) -> (w4477:T11[])
            n1952 = Reverse 1D Array(array=w4477) -> (reversed array=w4478:T11[])
            n1953 = for {
              tunnel: [w4494] -> w4488 mode=indexing
              tunnel: w4487 -> [w4493]
              tunnel: w4478 -> [w4492] mode=indexing
              n1954 = Unbundle By Name(w4492) -> ("command"=w4491:string, "command data"=w4490:variant)
              n1955 = call "App enquece.vi"("Priority Enquece"=TRUE, "command data"=w4490, "command"=w4491, "queue in"=w4493) -> ("error out"=w4494:errorcluster)  [unwired: 6 in, 1 out]
            }
          }
          frame True {
          }
        }
        n1956 = Merge Errors(w4466, w4468) -> (w4467:errorcluster)
      }
      frame "Test DRV 32" {
        w4501 = 32  # DUT index(0-59)
        n1957 = disable-structure shown="LOGGING==TRUE" {
          disable-tunnel: w4502 -> [w4537 _]
          frame condition #0 (active) {
            n1958 = Empty String/Path?(string/path=w4537) -> (empty?=w4540:bool)
            n1959 = Select(t="Quece timeout", s=w4540, f=w4537) -> (s? t:f=w4536:string)
            n1960 = call "string log (SubVI).vi"("Enum"=enum16{"Init", "Log", "Read"}."Log", "state Name"=w4536) -> ()  [unwired: 8 in, 2 out]
          }
          frame condition #1 {
          }
        }
        n1961 = call "progress string(SubVI).vi"("String 3"=w4502, "String in"=w4503) -> ("String out"=w4504:string)  [unwired: 9 in]
        n1962 = call "FGV Driver Data.vi"("DUT index(1-60)"=w4501) -> ("DUT SC"=w4500:bool)  [unwired: 7 in, 3 out]
        n1963 = case shown="False" w4500 {
          tunnel: [w4529 _] -> w4509
          tunnel: w4506 -> [w4528 _]
          frame False {
            w4516 = T11 {"command"="", "command data"=variant} ("element")
            w4515 = "MEAS.mux6_1"
            n1964 = To Variant(anything=T4."mux6-1_channel0" ("mux6_1(3wires)_encode")) -> (Variant=w4514:variant)
            n1965 = To Variant(anything=T4."mux6_1_channel2_3" ("mux6_1(3wires)_encode")) -> (Variant=w4526:variant)
            n1966 = To Variant(anything=T4."mux6_1_channel2_2" ("mux6_1(3wires)_encode")) -> (Variant=w4524:variant)
            n1967 = Bundle By Name(cluster=w4516, "command"=w4515, "command data"=w4524) -> (w4523:T11)
            n1968 = Bundle By Name(cluster=w4516, "command"=w4515, "command data"=w4526) -> (w4522:T11)
            n1969 = Bundle By Name(cluster=w4516, "command"=w4515, "command data"=w4514) -> ()  [unwired: 1 out]
            n1970 = Bundle By Name(cluster=w4516, "command"="MEAS.DMM dual read") -> (w4520:T11)
            n1971 = Build Array(w4523, w4522, w4520) -> (w4518:T11[])
            n1972 = Reverse 1D Array(array=w4518) -> (reversed array=w4519:T11[])
            n1973 = for {
              tunnel: [w4535] -> w4529 mode=indexing
              tunnel: w4528 -> [w4534]
              tunnel: w4519 -> [w4533] mode=indexing
              n1974 = Unbundle By Name(w4533) -> ("command"=w4532:string, "command data"=w4531:variant)
              n1975 = call "App enquece.vi"("Priority Enquece"=TRUE, "command data"=w4531, "command"=w4532, "queue in"=w4534) -> ("error out"=w4535:errorcluster)  [unwired: 6 in, 1 out]
            }
          }
          frame True {
          }
        }
        n1976 = Merge Errors(w4507, w4509) -> (w4508:errorcluster)
      }
      frame "Test DRV 33" {
        w4542 = 33  # DUT index(0-59)
        n1977 = disable-structure shown="LOGGING==TRUE" {
          disable-tunnel: w4543 -> [w4578 _]
          frame condition #0 (active) {
            n1978 = Empty String/Path?(string/path=w4578) -> (empty?=w4581:bool)
            n1979 = Select(t="Quece timeout", s=w4581, f=w4578) -> (s? t:f=w4577:string)
            n1980 = call "string log (SubVI).vi"("Enum"=enum16{"Init", "Log", "Read"}."Log", "state Name"=w4577) -> ()  [unwired: 8 in, 2 out]
          }
          frame condition #1 {
          }
        }
        n1981 = call "progress string(SubVI).vi"("String 3"=w4543, "String in"=w4544) -> ("String out"=w4545:string)  [unwired: 9 in]
        n1982 = call "FGV Driver Data.vi"("DUT index(1-60)"=w4542) -> ("DUT SC"=w4541:bool)  [unwired: 7 in, 3 out]
        n1983 = case shown="False" w4541 {
          tunnel: [w4570 _] -> w4550
          tunnel: w4547 -> [w4569 _]
          frame False {
            w4557 = T11 {"command"="", "command data"=variant} ("element")
            w4556 = "MEAS.mux6_1"
            n1984 = To Variant(anything=T4."mux6-1_channel0" ("mux6_1(3wires)_encode")) -> (Variant=w4555:variant)
            n1985 = To Variant(anything=T4."mux6_1_channel3_3" ("mux6_1(3wires)_encode")) -> (Variant=w4567:variant)
            n1986 = To Variant(anything=T4."mux6_1_channel3_2" ("mux6_1(3wires)_encode")) -> (Variant=w4565:variant)
            n1987 = Bundle By Name(cluster=w4557, "command"=w4556, "command data"=w4565) -> (w4564:T11)
            n1988 = Bundle By Name(cluster=w4557, "command"=w4556, "command data"=w4567) -> (w4563:T11)
            n1989 = Bundle By Name(cluster=w4557, "command"=w4556, "command data"=w4555) -> ()  [unwired: 1 out]
            n1990 = Bundle By Name(cluster=w4557, "command"="MEAS.DMM dual read") -> (w4561:T11)
            n1991 = Build Array(w4564, w4563, w4561) -> (w4559:T11[])
            n1992 = Reverse 1D Array(array=w4559) -> (reversed array=w4560:T11[])
            n1993 = for {
              tunnel: [w4576] -> w4570 mode=indexing
              tunnel: w4569 -> [w4575]
              tunnel: w4560 -> [w4574] mode=indexing
              n1994 = Unbundle By Name(w4574) -> ("command"=w4573:string, "command data"=w4572:variant)
              n1995 = call "App enquece.vi"("Priority Enquece"=TRUE, "command data"=w4572, "command"=w4573, "queue in"=w4575) -> ("error out"=w4576:errorcluster)  [unwired: 6 in, 1 out]
            }
          }
          frame True {
          }
        }
        n1996 = Merge Errors(w4548, w4550) -> (w4549:errorcluster)
      }
      frame "Test DRV 34" {
        w4583 = 34  # DUT index(0-59)
        n1997 = disable-structure shown="LOGGING==TRUE" {
          disable-tunnel: w4584 -> [w4619 _]
          frame condition #0 (active) {
            n1998 = Empty String/Path?(string/path=w4619) -> (empty?=w4622:bool)
            n1999 = Select(t="Quece timeout", s=w4622, f=w4619) -> (s? t:f=w4618:string)
            n2000 = call "string log (SubVI).vi"("Enum"=enum16{"Init", "Log", "Read"}."Log", "state Name"=w4618) -> ()  [unwired: 8 in, 2 out]
          }
          frame condition #1 {
          }
        }
        n2001 = call "progress string(SubVI).vi"("String 3"=w4584, "String in"=w4585) -> ("String out"=w4586:string)  [unwired: 9 in]
        n2002 = call "FGV Driver Data.vi"("DUT index(1-60)"=w4583) -> ("DUT SC"=w4582:bool)  [unwired: 7 in, 3 out]
        n2003 = case shown="False" w4582 {
          tunnel: [w4611 _] -> w4591
          tunnel: w4588 -> [w4610 _]
          frame False {
            w4598 = T11 {"command"="", "command data"=variant} ("element")
            w4597 = "MEAS.mux6_1"
            n2004 = To Variant(anything=T4."mux6-1_channel0" ("mux6_1(3wires)_encode")) -> (Variant=w4596:variant)
            n2005 = To Variant(anything=T4."mux6_1_channel4_3" ("mux6_1(3wires)_encode")) -> (Variant=w4608:variant)
            n2006 = To Variant(anything=T4."mux6_1_channel4_2" ("mux6_1(3wires)_encode")) -> (Variant=w4606:variant)
            n2007 = Bundle By Name(cluster=w4598, "command"=w4597, "command data"=w4606) -> (w4605:T11)
            n2008 = Bundle By Name(cluster=w4598, "command"=w4597, "command data"=w4608) -> (w4604:T11)
            n2009 = Bundle By Name(cluster=w4598, "command"=w4597, "command data"=w4596) -> ()  [unwired: 1 out]
            n2010 = Bundle By Name(cluster=w4598, "command"="MEAS.DMM dual read") -> (w4602:T11)
            n2011 = Build Array(w4605, w4604, w4602) -> (w4600:T11[])
            n2012 = Reverse 1D Array(array=w4600) -> (reversed array=w4601:T11[])
            n2013 = for {
              tunnel: [w4617] -> w4611 mode=indexing
              tunnel: w4610 -> [w4616]
              tunnel: w4601 -> [w4615] mode=indexing
              n2014 = Unbundle By Name(w4615) -> ("command"=w4614:string, "command data"=w4613:variant)
              n2015 = call "App enquece.vi"("Priority Enquece"=TRUE, "command data"=w4613, "command"=w4614, "queue in"=w4616) -> ("error out"=w4617:errorcluster)  [unwired: 6 in, 1 out]
            }
          }
          frame True {
          }
        }
        n2016 = Merge Errors(w4589, w4591) -> (w4590:errorcluster)
      }
      frame "Test DRV 35" {
        w4624 = 35  # DUT index(0-59)
        n2017 = disable-structure shown="LOGGING==TRUE" {
          disable-tunnel: w4625 -> [w4660 _]
          frame condition #0 (active) {
            n2018 = Empty String/Path?(string/path=w4660) -> (empty?=w4663:bool)
